vi "Write TRC.vi"(1 "Frame":i32, 2 "Unidentified Data":sgl[](array[numeric]), 3 "Marker Data":sgl[][](array[numeric]), 4 "Markers":string[](array[string])) -> ()   [LabVIEW 2010]
uses:
  <vilib>/Utility/file.llb/Write To Spreadsheet File (string).vi
  <vilib>/Utility/file.llb/Write To Spreadsheet File (DBL).vi
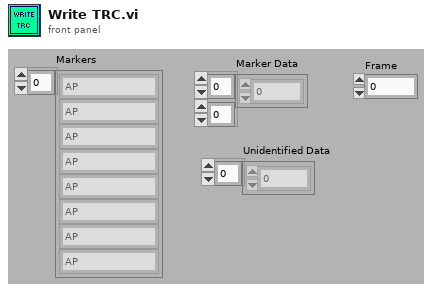
[diagram p1: front panel]
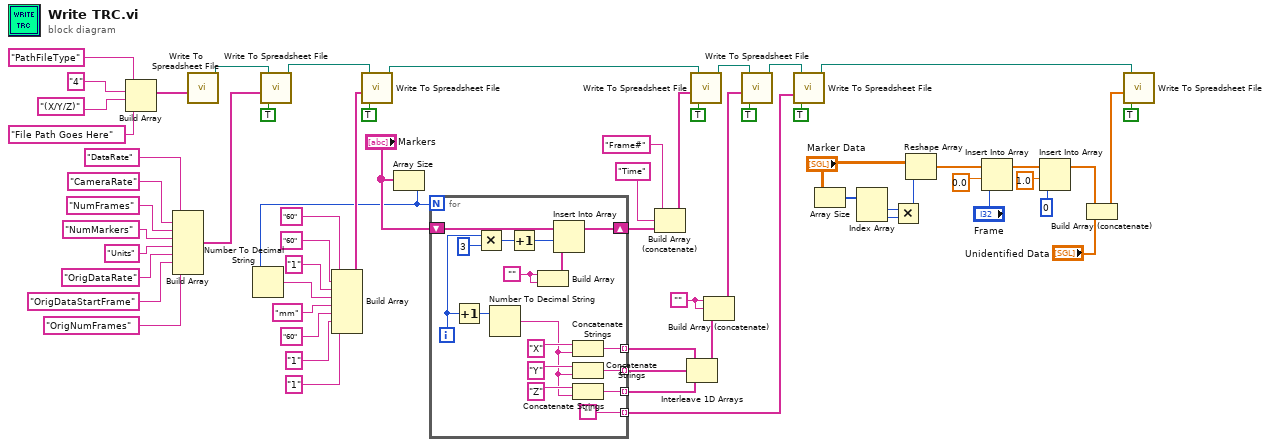
[diagram p0: block diagram]
diagram:
  w16 = ""
  n1 = Build Array("PathFileType", "4", "(X/Y/Z)", "File Path Goes Here") -> (w58:string[])
  n2 = Build Array("DataRate", "CameraRate", "NumFrames", "NumMarkers", "Units", "OrigDataRate", "OrigDataStartFrame", "OrigNumFrames") -> (w47:string[])
  n3 = call-poly <vilib>:"Write To Spreadsheet File.vi"("1D data"=w58) -> ("new file path (Not A Path if cancelled)"=w57:path)  [unwired: 7 in]
  n4 = call-poly <vilib>:"Write To Spreadsheet File.vi"("append to file? (new file:F)"=TRUE, "1D data"=w47, "file path (dialog if empty)"=w57) -> ("new file path (Not A Path if cancelled)"=w46:path)  [unwired: 5 in]
  n5 = Array Size(array="Markers") -> (size(s)=w18:i32)
  n6 = Number To Decimal String(number=w18) -> (decimal integer string=w17:string)  [unwired: 1 in]
  n7 = Build Array("60", "60", "1", w17, "mm", "60", "1", "1") -> (w37:string[])
  n8 = call-poly <vilib>:"Write To Spreadsheet File.vi"("append to file? (new file:F)"=TRUE, "1D data"=w37, "file path (dialog if empty)"=w46) -> ("new file path (Not A Path if cancelled)"=w35:path)  [unwired: 5 in]
  n9 = for {
    N: w18 -> [_]
    tunnel: [w72] -> w31 mode=indexing
    tunnel: [w71] -> w30 mode=indexing
    tunnel: [w70] -> w29 mode=indexing
    shift-right: [w68] -> w23
    shift-left: "Markers" -> [w79]
    tunnel: [""] -> w20 mode=indexing
    i -> [w64]
    w65 = ""
    n10 = Increment(x=w64) -> (x+1=w76:i32)
    n11 = Multiply(x=w64, y=3 ("x")) -> (x*y=w69:i32)
    n12 = Number To Decimal String(number=w76) -> (decimal integer string=w73:string)  [unwired: 1 in]
    n13 = Increment(x=w69) -> (x+1=w67:i32)
    n14 = Build Array(w65, w65) -> (w78:string[])
    n15 = Insert Into Array(array=w79, index=w67, new element=w78) -> (w68:string[])
    n16 = Concatenate Strings("X", w73) -> (w72:string)
    n17 = Concatenate Strings("Y", w73) -> (w71:string)
    n18 = Concatenate Strings("Z", w73) -> (w70:string)
  }
  n19 = Build Array (concatenate)("Frame#", "Time", w23) -> (w32:string[])
  n20 = Interleave 1D Arrays(w31, w30, w29) -> (w25:string[])
  n21 = call-poly <vilib>:"Write To Spreadsheet File.vi"("append to file? (new file:F)"=TRUE, "1D data"=w32, "file path (dialog if empty)"=w35) -> ("new file path (Not A Path if cancelled)"=w27:path)  [unwired: 5 in]
  n22 = Build Array (concatenate)(w16, w16, w25) -> (w24:string[])
  n23 = call-poly <vilib>:"Write To Spreadsheet File.vi"("append to file? (new file:F)"=TRUE, "1D data"=w24, "file path (dialog if empty)"=w27) -> ("new file path (Not A Path if cancelled)"=w21:path)  [unwired: 5 in]
  n24 = call-poly <vilib>:"Write To Spreadsheet File.vi"("append to file? (new file:F)"=TRUE, "1D data"=w20, "file path (dialog if empty)"=w21) -> ("new file path (Not A Path if cancelled)"=w19:path)  [unwired: 5 in]
  n25 = Array Size(array="Marker Data") -> (size(s)=w9:i32[])
  n26 = Index Array(array=w9) -> (element #1=w8:i32, element #2=w7:i32)  [unwired: 2 in]
  n27 = Multiply(x=w8, y=w7) -> (x*y=w5:i32)
  n28 = Reshape Array("Marker Data", w5) -> (w4:sgl[])
  n29 = Insert Into Array(array=w4, index=0.0 ("new element/subarray"), new element="Frame") -> (w14:sgl[])
  n30 = Insert Into Array(array=w14, index=1.0 ("new element/subarray"), new element=0 ("disabled index (col)")) -> (w2:sgl[])
  n31 = Build Array (concatenate)(w2, "Unidentified Data") -> (w1:sgl[])
  n32 = call-poly <vilib>:"Write To Spreadsheet File.vi"("append to file? (new file:F)"=TRUE, "1D data"=w1, "file path (dialog if empty)"=w19) -> ()  [unwired: 5 in, 1 out]
